vi "TorqueCurrentFOC Setter.vi"(0 "DeviceReference":T1, 1 "Deadband":dbl, 2 "LimitForwardMotion":bool, 3 "Update Frequency (Hz)":dbl=100.0, 5 "StopSendingOtherRequests":bool=TRUE, 7 "Output":dbl, 9 "MaxAbsDutyCycle":dbl=1.0, 12 "OverrideCoastDurNeutral":bool, 13 "LimitReverseMotion":bool) -> (4 "DeviceReference Out":T1)   [LabVIEW 2023]
doc: "Request a specified motor current (field oriented control).\nThis control request will drive the motor to the requested motor (stator) current value. This leverages field oriented control (FOC), which means greater peak power than what is documented. This scales to torque based on Motor's kT constant."
uses:
  Users/Cory/Documents/PhoenixPro-LabVIEW-Generation/controls/DeviceReference.ctl
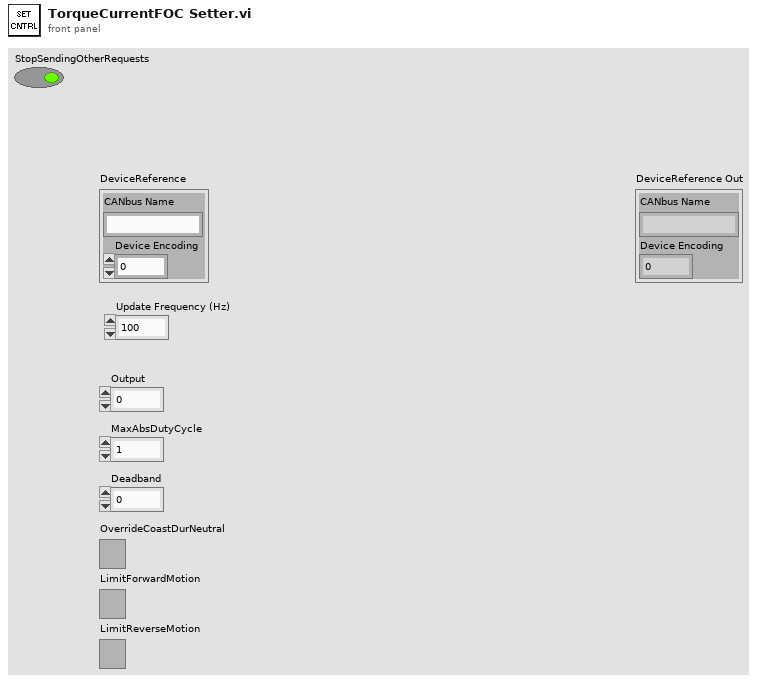
[diagram p1: front panel]
types:
  T1 = typedef "DeviceReference.ctl" = cluster{"CANbus Name":string, "Device Encoding":u32}
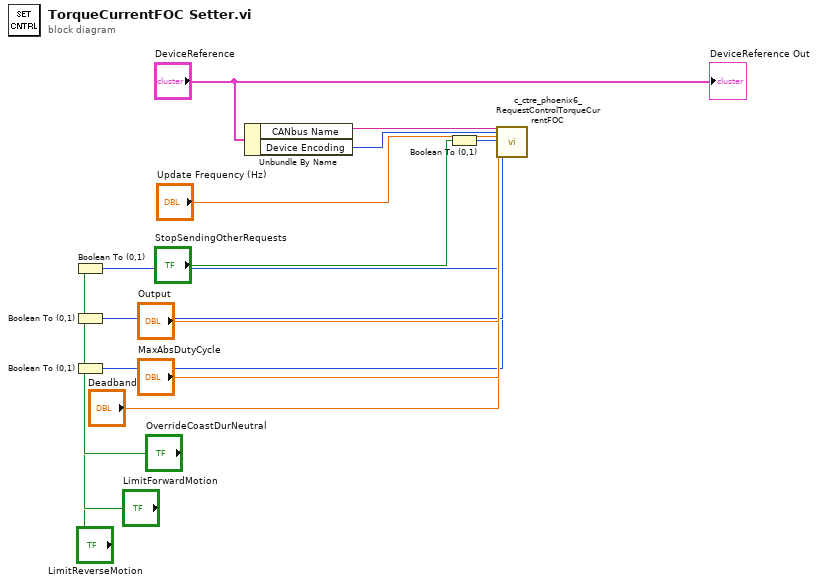
[diagram p0: block diagram]
diagram:
  n1 = Boolean To (0,1)(Boolean="OverrideCoastDurNeutral") -> (0, 1=w5:i16)
  n2 = Boolean To (0,1)(Boolean="LimitForwardMotion") -> (0, 1=w3:i16)
  n3 = Boolean To (0,1)(Boolean="LimitReverseMotion") -> (0, 1=w1:i16)
  n4 = Unbundle By Name("DeviceReference") -> ("CANbus Name"=w14:string, "Device Encoding"=w13:u32)
  n5 = Boolean To (0,1)(Boolean="StopSendingOtherRequests") -> (0, 1=w10:i16)
  n6 = call <vilib>:"c_ctre_phoenix6_RequestControlTorqueCurrentFOC.vi"("String"=w14, "Numeric 2"=w13, "Numeric 3"="Update Frequency (Hz)", "Numeric 4"=w10, "Numeric 5"="Output", "Numeric 6"="MaxAbsDutyCycle", "Numeric 7"="Deadband", "Numeric 8"=w5, "Numeric 9"=w3, "Numeric 10"=w1) -> ()  [unwired: 17 in, 1 out]
  "DeviceReference Out" <- "DeviceReference"
